vi "Time-interpolated virtual calibration generator.vi"(1 "time fraction (0...1)":dbl=0.5 min=0.0 max=1.0, 2 "t1* Calibration data":T1, 3 "t0 Calibration data":T1) -> (0 "t_frac Calibration data":T1)   [LabVIEW 2022 SP3]
uses:
  Ctls/Calibration data.ctl
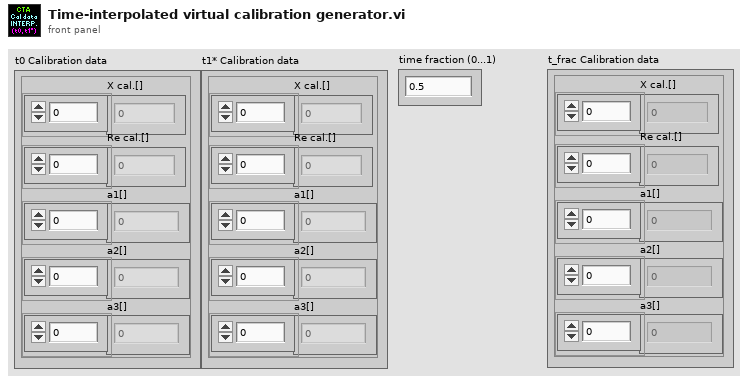
[diagram p1: front panel]
types:
  T1 = typedef "Calibration data.ctl" = cluster{"X cal.[]":dbl[], "Re cal.[]":dbl[], "a1[]":dbl[], "a2[]":dbl[], "a3[]":dbl[]}
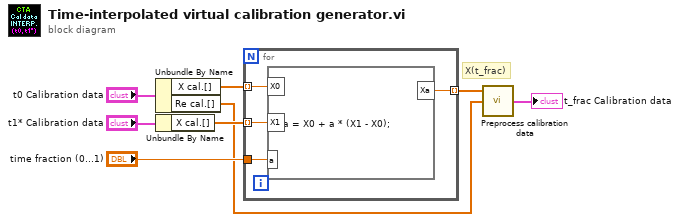
[diagram p0: block diagram]
diagram:
  # "X(t_frac)"
  n1 = Unbundle By Name("t0 Calibration data") -> ("X cal.[]"=w5:dbl[], "Re cal.[]"=w2:dbl[])
  n2 = Unbundle By Name("t1* Calibration data") -> ("X cal.[]"=w7:dbl[])
  n3 = for {
    tunnel: w7 -> [w12] mode=indexing
    tunnel: "time fraction (0...1)" -> [w10]
    tunnel: w5 -> [w11] mode=indexing
    tunnel: [w9] -> w3 mode=indexing
    n4 = formula code="Xa = X0 + a * (X1 - X0);"("a"=w10, "X0"=w11, "X1"=w12) -> ("Xa"=w9:dbl)
  }
  n5 = call "Preprocess calibration data.vi"("Re cal.[]"=w2, "X cal.[]"=w3) -> ("Calibration data"=→"t_frac Calibration data":T1)  [unwired: 1 in]
